vi "Configure Acquisition Time.vi"(8 "error in (no error)":errorcluster, 10 "acquisition time, ms":u16(ring) items=["4.08", "6.08", "12.20", "20.96", "42.61", "85.20", "170.40", "348.60", "687.20"], 11 "VI Probe in":refnum<class "PL MKS VI Probe.lvclass">) -> (0 "error out":errorcluster, 3 "VI Probe out":refnum<class "PL MKS VI Probe.lvclass">)   [LabVIEW 2015, in "PL MKS VI Probe.lvclass"]
doc: "Configures acquisition time."
uses:
  PL MKS VI Probe.lvclass
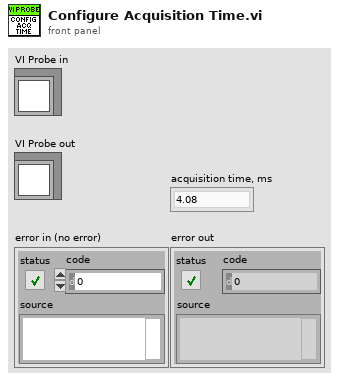
[diagram p1: front panel]
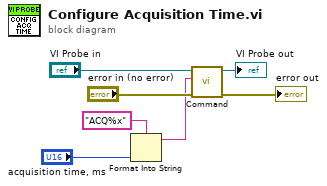
[diagram p0: block diagram]
diagram:
  n1 = Format Into String(format string="ACQ%x", "acquisition time, ms") -> (resulting string=w2:string)  [unwired: 2 in, 1 out]
  n2 = call "Command.vi"("error in (no error)"="error in (no error)", "command"=w2, "VI Probe in"="VI Probe in") -> ("error out"=→"error out":errorcluster, "VI Probe out"=→"VI Probe out":refnum<class "PL MKS VI Probe.lvclass">)  [unwired: 6 in, 1 out]
